vi "Lab Panel V4.83.vi"() -> ()   [LabVIEW 2013] (continued)
                n1623 = property on="SET LAB03-2" class="Clust (strict)"("DisabledEnum"=w2555) -> ()  [unwired: 2 in, 2 out]
                n1624 = property on="SET LAB04-1" class="Clust (strict)"("DisabledEnum"=w2554) -> ()  [unwired: 2 in, 2 out]
                n1625 = property on="SET LAB04-2" class="Clust (strict)"("DisabledEnum"=w2553) -> ()  [unwired: 2 in, 2 out]
                n1626 = property on="O/I  LAB05-2" class="Bool (strict)"("DisabledEnum"=w2551) -> ()  [unwired: 2 in, 2 out]
                n1627 = property on="O/I  LAB05-1" class="Bool (strict)"("DisabledEnum"=w2552) -> ()  [unwired: 2 in, 2 out]
                n1628 = property on="O/I  LAB04-1" class="Bool (strict)"("DisabledEnum"=w2554) -> ()  [unwired: 2 in, 2 out]
                n1629 = property on="O/I  LAB04-2" class="Bool (strict)"("DisabledEnum"=w2553) -> ()  [unwired: 2 in, 2 out]
                n1630 = property on="O/I  LAB03-2" class="Bool (strict)"("DisabledEnum"=w2555) -> ()  [unwired: 2 in, 2 out]
                n1631 = Not(x=w2560) -> (.not. x?=w2561:bool)
                n1632 = Not(x=w2559) -> (.not. x?=w2562:bool)
                n1633 = Not(x=w2558) -> (.not. x?=w2563:bool)
                n1634 = property on="RESULT LAB05-2" class="Bool (strict)"("Visible"=w2561) -> ()  [unwired: 2 in, 2 out]
                n1635 = property on="RESULT LAB05-1" class="Bool (strict)"("Visible"=w2562) -> ()  [unwired: 2 in, 2 out]
                n1636 = Not(x=w2557) -> (.not. x?=w2564:bool)
                n1637 = property on="RESULT LAB04-2" class="Bool (strict)"("Visible"=w2563) -> ()  [unwired: 2 in, 2 out]
                n1638 = Not(x=w2556) -> (.not. x?=w2565:bool)
                n1639 = property on="RESULT LAB04-1" class="Bool (strict)"("Visible"=w2564) -> ()  [unwired: 2 in, 2 out]
                n1640 = property on="RESULT LAB03-2" class="Bool (strict)"("Visible"=w2565) -> ()  [unwired: 2 in, 2 out]
              }
              frame #2 {
                # "disable calibrate if any test running"
                n1641 = Or(x=w2588, y=w2587) -> (x .or. y?=w2581:bool)
                n1642 = Or(x=w2590, y=w2589) -> (x .or. y?=w2583:bool)
                n1643 = Or(x=w2594, y=w2593) -> (x .or. y?=w2585:bool)
                n1644 = Or(x=w2592, y=w2591) -> (x .or. y?=w2584:bool)
                n1645 = Or(x=w2596, y=w2595) -> (x .or. y?=w2586:bool)
                n1646 = Or(x=w2584, y=w2583) -> (x .or. y?=w2582:bool)
                n1647 = Or(x=w2586, y=w2585) -> (x .or. y?=w2580:bool)
                n1648 = Or(x=w2582, y=w2581) -> (x .or. y?=w2579:bool)
                n1649 = Or(x=w2580, y=w2579) -> (x .or. y?=w2578:bool)
                n1650 = case shown="False" w2578 {
                  tunnel: [0 2] -> w2577
                  frame False {
                  }
                  frame True {
                  }
                }
                n1651 = property on="JIG TEST" class="Clust (strict)"("DisabledEnum"=w2577) -> ()  [unwired: 2 in, 2 out]
                n1652 = property on="Network Directory" class="Path"("DisabledEnum"=w2577) -> ()  [unwired: 2 in, 2 out]
                n1653 = property on="MAIL SETTINGS" class="Clust (strict)"("DisabledEnum"=w2577) -> ()  [unwired: 2 in, 2 out]
                n1654 = property on="SET (cal)" class="Bool (strict)"("DisabledEnum"=w2577) -> ()  [unwired: 2 in, 2 out]
                n1655 = property on="ADMIN" class="Bool (strict)"("DisabledEnum"=0) -> ()  [unwired: 2 in, 2 out]
              }
            }
          }
          frame #8 {
            # "drive jigs"
            n1656 = stacked-sequence {
              frame #0 {
                # "jig on"
                n1657 = local read "jig cycle"() -> (w2604:dbl)
                n1658 = property on="JIG TEST" class="Clust (strict)"() -> ("DisabledEnum"=w2601:T14)  [unwired: 2 in, 2 out]
                n1659 = Equal?(x=w2601, y=2) -> (x = y?=w2600:bool)
                n1660 = Equal?(x=w2604, y=0) -> (x = y?=w2602:bool)
                n1661 = And(x=w2602, y=w2600) -> (x .and. y?=w2599:bool)
                n1662 = case shown="True" w2599 {
                  frame False {
                  }
                  frame True {
                    n1663 = local read "run lab01-1"() -> (w2615:bool)
                    n1664 = local read "run lab01-2"() -> (w2614:bool)
                    n1665 = local read "run lab02-1"() -> (w2613:bool)
                    n1666 = local read "run lab02-2"() -> (w2612:bool)
                    n1667 = local read "run lab03-1"() -> (w2611:bool)
                    n1668 = local read "run lab03-2"() -> (w2610:bool)
                    n1669 = local read "run lab04-1"() -> (w2609:bool)
                    n1670 = local read "run lab04-2"() -> (w2608:bool)
                    n1671 = local read "run lab05-1"() -> (w2607:bool)
                    n1672 = local read "run lab05-2"() -> (w2606:bool)
                    n1673 = local write "JIG LAB03-2"(w2610) -> ()
                    n1674 = local write "JIG LAB01-1"(w2615) -> ()
                    n1675 = local write "JIG LAB01-2"(w2614) -> ()
                    n1676 = local write "JIG LAB02-1"(w2613) -> ()
                    n1677 = local write "JIG LAB02-2"(w2612) -> ()
                    n1678 = local write "JIG LAB03-1"(w2611) -> ()
                    n1679 = local write "JIG LAB04-1"(w2609) -> ()
                    n1680 = local write "JIG LAB04-2"(w2608) -> ()
                    n1681 = local write "JIG LAB05-1"(w2607) -> ()
                    n1682 = local write "JIG LAB05-2"(w2606) -> ()
                  }
                }
              }
              frame #1 {
                # "jig off"
                n1683 = local read "jig cycle"() -> (w2622:dbl)
                n1684 = local read "on loops"() -> (w2621:dbl)
                n1685 = property on="JIG TEST" class="Clust (strict)"() -> ("DisabledEnum"=w2620:T14)  [unwired: 2 in, 2 out]
                n1686 = Equal?(x=w2620, y=2) -> (x = y?=w2618:bool)
                n1687 = Equal?(x=w2622, y=w2621) -> (x = y?=w2617:bool)
                n1688 = And(x=w2617, y=w2618) -> (x .and. y?=w2616:bool)
                n1689 = case shown="True" w2616 {
                  frame False {
                  }
                  frame True {
                    w2673 = FALSE
                    w2674 = TRUE
                    w2672 = 2
                    n1690 = local read "SELECT LAB05-2"() -> (w2663:T3)
                    n1691 = local read "SELECT LAB04-2"() -> (w2665:T3)
                    n1692 = local read "SELECT LAB04-1"() -> (w2666:T3)
                    n1693 = local read "SELECT LAB05-1"() -> (w2664:T3)
                    n1694 = local read "SELECT LAB03-2"() -> (w2667:T3)
                    n1695 = local read "SELECT LAB02-1"() -> (w2670:T3)
                    n1696 = local read "SELECT LAB03-1"() -> (w2668:T3)
                    n1697 = local read "SELECT LAB02-2"() -> (w2669:T3)
                    n1698 = local read "SELECT LAB01-2"() -> (w2671:T3)
                    n1699 = local read "run lab05-1"() -> (w2633:bool)
                    n1700 = local read "run lab05-2"() -> (w2632:bool)
                    n1701 = local read "SELECT LAB01-1"() -> (w2675:T3)
                    n1702 = local read "run lab04-2"() -> (w2634:bool)
                    n1703 = local read "run lab04-1"() -> (w2635:bool)
                    n1704 = local read "run lab01-1"() -> (w2651:bool)
                    n1705 = local read "run lab01-2"() -> (w2640:bool)
                    n1706 = local read "run lab03-2"() -> (w2636:bool)
                    n1707 = local read "run lab03-1"() -> (w2637:bool)
                    n1708 = local read "run lab02-1"() -> (w2639:bool)
                    n1709 = local read "run lab02-2"() -> (w2638:bool)
                    n1710 = Equal?(x=w2672, y=w2668) -> (x = y?=w2646:bool)
                    n1711 = Equal?(x=w2672, y=w2667) -> (x = y?=w2645:bool)
                    n1712 = Equal?(x=w2672, y=w2666) -> (x = y?=w2644:bool)
                    n1713 = Equal?(x=w2672, y=w2665) -> (x = y?=w2643:bool)
                    n1714 = Equal?(x=w2672, y=w2664) -> (x = y?=w2642:bool)
                    n1715 = Equal?(x=w2672, y=w2663) -> (x = y?=w2641:bool)
                    n1716 = Equal?(x=w2672, y=w2675) -> (x = y?=w2652:bool)
                    n1717 = Equal?(x=w2672, y=w2670) -> (x = y?=w2648:bool)
                    n1718 = Equal?(x=w2672, y=w2669) -> (x = y?=w2647:bool)
                    n1719 = Equal?(x=w2672, y=w2671) -> (x = y?=w2649:bool)
                    n1720 = And(x=w2643, y=w2634) -> (x .and. y?=w2625:bool)
                    n1721 = And(x=w2646, y=w2637) -> (x .and. y?=w2628:bool)
                    n1722 = And(x=w2644, y=w2635) -> (x .and. y?=w2626:bool)
                    n1723 = And(x=w2641, y=w2632) -> (x .and. y?=w2623:bool)
                    n1724 = And(x=w2647, y=w2638) -> (x .and. y?=w2629:bool)
                    n1725 = And(x=w2645, y=w2636) -> (x .and. y?=w2627:bool)
                    n1726 = And(x=w2642, y=w2633) -> (x .and. y?=w2624:bool)
                    n1727 = And(x=w2649, y=w2640) -> (x .and. y?=w2631:bool)
                    n1728 = And(x=w2652, y=w2651) -> (x .and. y?=w2650:bool)
                    n1729 = And(x=w2648, y=w2639) -> (x .and. y?=w2630:bool)
                    n1730 = Select(t=w2674, s=w2650, f=w2673) -> (s? t:f=w2653:bool)
                    n1731 = Select(t=w2674, s=w2631, f=w2673) -> (s? t:f=w2654:bool)
                    n1732 = Select(t=w2674, s=w2630, f=w2673) -> (s? t:f=w2655:bool)
                    n1733 = Select(t=w2674, s=w2629, f=w2673) -> (s? t:f=w2656:bool)
                    n1734 = Select(t=w2674, s=w2628, f=w2673) -> (s? t:f=w2657:bool)
                    n1735 = Select(t=w2674, s=w2627, f=w2673) -> (s? t:f=w2658:bool)
                    n1736 = Select(t=w2674, s=w2626, f=w2673) -> (s? t:f=w2659:bool)
                    n1737 = Select(t=w2674, s=w2625, f=w2673) -> (s? t:f=w2660:bool)
                    n1738 = Select(t=w2674, s=w2624, f=w2673) -> (s? t:f=w2661:bool)
                    n1739 = Select(t=w2674, s=w2623, f=w2673) -> (s? t:f=w2662:bool)
                    n1740 = local write "JIG LAB03-2"(w2658) -> ()
                    n1741 = local write "JIG LAB02-1"(w2655) -> ()
                    n1742 = local write "JIG LAB02-2"(w2656) -> ()
                    n1743 = local write "JIG LAB01-2"(w2654) -> ()
                    n1744 = local write "JIG LAB03-1"(w2657) -> ()
                    n1745 = local write "JIG LAB01-1"(w2653) -> ()
                    n1746 = local write "JIG LAB05-2"(w2662) -> ()
                    n1747 = local write "JIG LAB04-1"(w2659) -> ()
                    n1748 = local write "JIG LAB05-1"(w2661) -> ()
                    n1749 = local write "JIG LAB04-2"(w2660) -> ()
                  }
                }
              }
            }
          }
          frame #9 {
            # "enable  jig test output if no test busy"
            n1750 = property on="JIG TEST" class="Clust (strict)"() -> ("DisabledEnum"=w2678:T14)  [unwired: 2 in, 2 out]
            n1751 = Equal?(x=w2678, y=0) -> (x = y?=w2676:bool)
            n1752 = case shown="True" w2676 {
              frame False {
              }
              frame True {
                n1753 = local read "JIG TEST"() -> (w2689:T9)
                n1754 = Unbundle(w2689) -> ("LAB01-1"=w2688:bool, "LAB01-2"=w2687:bool, "LAB02-1"=w2686:bool, "LAB02-2"=w2685:bool, "LAB03-1"=w2684:bool, "LAB03-2"=w2683:bool, "LAB04-1"=w2682:bool, "LAB04-2"=w2681:bool, "LAB05-1"=w2680:bool, "LAB05-2"=w2679:bool)
                n1755 = local write "JIG LAB05-1"(w2680) -> ()
                n1756 = local write "JIG LAB05-2"(w2679) -> ()
                n1757 = local write "JIG LAB04-1"(w2682) -> ()
                n1758 = local write "JIG LAB04-2"(w2681) -> ()
                n1759 = local write "JIG LAB03-2"(w2683) -> ()
                n1760 = local write "JIG LAB01-1"(w2688) -> ()
                n1761 = local write "JIG LAB02-1"(w2686) -> ()
                n1762 = local write "JIG LAB03-1"(w2684) -> ()
                n1763 = local write "JIG LAB01-2"(w2687) -> ()
                n1764 = local write "JIG LAB02-2"(w2685) -> ()
              }
            }
          }
          frame #10 {
            # "drive digital output"
            n1765 = local read "O/I  LAB05-2"() -> (w2696:bool)
            n1766 = local read "O/I  LAB05-1"() -> (w2698:bool)
            n1767 = local read "JIG LAB05-2"() -> (w2695:bool)
            n1768 = local read "O/I  LAB04-2"() -> (w2700:bool)
            n1769 = local read "JIG LAB05-1"() -> (w2697:bool)
            n1770 = local read "JIG LAB04-2"() -> (w2699:bool)
            n1771 = local read "O/I  LAB03-1"() -> (w2705:bool)
            n1772 = local read "O/I  LAB04-1"() -> (w2701:bool)
            n1773 = local read "O/I  LAB02-1"() -> (w2709:bool)
            n1774 = local read "O/I  LAB02-2"() -> (w2707:bool)
            n1775 = local read "O/I  LAB03-2"() -> (w2703:bool)
            n1776 = local read "JIG LAB04-1"() -> (w2694:bool)
            n1777 = local read "JIG LAB03-2"() -> (w2702:bool)
            n1778 = local read "O/I  LAB01-2"() -> (w2711:bool)
            n1779 = local read "JIG LAB02-1"() -> (w2708:bool)
            n1780 = local read "JIG LAB02-2"() -> (w2706:bool)
            n1781 = local read "JIG LAB03-1"() -> (w2704:bool)
            n1782 = local read "O/I  LAB01-1"() -> (w2713:bool)
            n1783 = local read "JIG LAB01-2"() -> (w2710:bool)
            n1784 = local read "JIG LAB01-1"() -> (w2712:bool)
            n1785 = Build Array(w2700, w2699, w2698, w2697, w2696, w2695) -> (w2691:bool[])
            n1786 = Build Array(w2706, w2705, w2704, w2703, w2702, w2701, w2694) -> (w2692:bool[])
            n1787 = Build Array(w2713, w2712, w2711, w2710, w2709, w2708, w2707) -> (w2693:bool[])
            n1788 = local read "simulate"() -> (w2690:bool)
            n1789 = case shown="False" w2690 {
              tunnel: w2693 -> [w2716 _]
              tunnel: w2692 -> [w2715 _]
              tunnel: w2691 -> [w2714 _]
              frame False {
                n1790 = call "sub vi - Drive Relays All v6.vi"("Array #2"=w2714, "Array #1"=w2715, "Array #0"=w2716) -> ()  [unwired: 8 in, 1 out]
              }
              frame True {
              }
            }
          }
          frame #11 {
            # "get analog values"
            n1791 = local read "on loops"() -> (w2723:dbl)
            n1792 = local read "jig cycle"() -> (w2720:dbl)
            n1793 = Add(x=w2723, y=1) -> (x+y=w2721:dbl)
            n1794 = Equal?(x=w2720, y=1) -> (x = y?=w2718:bool)
            n1795 = Equal?(x=w2720, y=w2721) -> (x = y?=w2719:bool)
            n1796 = Or(x=w2718, y=w2719) -> (x .or. y?=w2717:bool)
            n1797 = case shown="True" w2717 {
              frame False {
              }
              frame True {
                n1798 = local read "simulate"() -> (w2727:bool)
                n1799 = case shown="False" w2727 {
                  tunnel: [w2743 errorcluster[] [] ("array ERROR")] -> w2735
                  tunnel: [w2742 0.3 ("Analog loop time")] -> w2734
                  tunnel: [w2741 dynamicdata[] [] ("array GRAPH")] -> w2733
                  tunnel: [w2740 w2745] -> w2732
                  tunnel: [w2739 w2745] -> w2731
                  tunnel: [w2738 w2745] -> w2730
                  tunnel: [w2737 w2745] -> w2729
                  tunnel: [w2736 w2745] -> w2728
                  frame False {
                    n1800 = call "sub vi - Read Analog All v8.vi"() -> ("Analog loop time"=w2742:dbl, "array GRAPH"=w2741:dynamicdata[], "LAB01"=w2740:T23, "LAB02"=w2739:T24, "LAB03"=w2738:T25, "LAB04"=w2737:T26, "array ERROR"=w2743:errorcluster[], "LAB05"=w2736:T27)  [unwired: 8 in]
                  }
                  frame True {
                    w2745 = T27 {"LAB05-1 (A)"=10.0, "LAB05-1 (V)"=220.0, "LAB05-1 (PF)"=0.5, "LAB05-2 (A)"=15.0, "LAB05-2 (V)"=225.0, "LAB05-2 (PF)"=0.6} ("LAB05")
                  }
                }
                n1801 = local read "simulate"() -> (w2726:bool)
                n1802 = stacked-sequence {
                  tunnel: w2735 -> [w2752 _ _ _ _ _]
                  tunnel: w2734 -> [w2751 _ _ _ _ _]
                  tunnel: w2733 -> [w2750 _ _ _ _ _]
                  tunnel: w2732 -> [_ w2799 _ _ _ _]
                  tunnel: w2731 -> [_ _ w2806 _ _ _]
                  tunnel: w2730 -> [_ _ _ w2835 _ _]
                  tunnel: w2729 -> [_ _ _ _ w2862 _]
                  tunnel: w2728 -> [_ _ _ _ _ w2891]
                  tunnel: w2726 -> [_ w2777 w2805 w2833 w2861 w2889]
                  tunnel: T12 {"1  (A) cal"=1.0, "1 (V) cal"=1.0, "1 (PF) cal"=1.0, "1 (TL) cal"=1.0, "1 (TN) cal"=1.0, "2 (A) cal"=1.0, "2 (V) cal"=1.0, "2 (PF) cal"=1.0, "2 (TL) cal"=1.0, "2 (TN) cal"=1.0} ("CAL LAB01") -> [_ w2776 w2804 w2832 w2860 w2888]
                  frame #0 {
                    n1803 = local write "AI"(TRUE) -> ()
                    n1804 = global write "Global 1.vi" "RATE(Hz)"("RATE (Hz)") -> ()
                    n1805 = global write "Global 1.vi" "SAMPLES"("SAMPLES") -> ()
                    n1806 = Index Array(array=w2750, index=6) -> (element=→"LAB04-1 (GRAPH)":dynamicdata)
                    n1807 = Index Array(array=w2750, index=7) -> (element=→"LAB04-2 (GRAPH)":dynamicdata)
                    n1808 = Index Array(array=w2750, index=9) -> (element=→"LAB05-2 (GRAPH)":dynamicdata)
                    n1809 = Index Array(array=w2750, index=8) -> (element=→"LAB05-1 (GRAPH)":dynamicdata)
                    n1810 = Index Array(array=w2750, index=5) -> (element=→"LAB03-2 (GRAPH)":dynamicdata)
                    n1811 = Index Array(array=w2750, index=0) -> (element=→"LAB01-1 (GRAPH)":dynamicdata)
                    n1812 = Index Array(array=w2750, index=1) -> (element=→"LAB01-2 (GRAPH)":dynamicdata)
                    n1813 = Index Array(array=w2750, index=2) -> (element=→"LAB02-1 (GRAPH)":dynamicdata)
                    n1814 = Index Array(array=w2750, index=3) -> (element=→"LAB02-2 (GRAPH)":dynamicdata)
                    n1815 = Index Array(array=w2750, index=4) -> (element=→"LAB03-1 (GRAPH)":dynamicdata)
                    "AI loop time" <- w2751
                    "Analog Error Array" <- w2752
                  }
                  frame #1 {
                    n1816 = Unbundle By Name(w2799) -> ("LAB05-1 (A)"=w2797:dbl, "LAB05-1 (V)"=w2796:dbl, "LAB05-1 (PF)"=w2795:dbl, "LAB05-2 (A)"=w2794:dbl, "LAB05-2 (V)"=w2793:dbl, "LAB05-2 (PF)"=w2792:dbl)
                    n1817 = case shown="False" w2777 {
                      tunnel: [w2800 w2801] -> w2798
                      tunnel: w2776 -> [_ w2801]
                      frame False {
                        n1818 = local read "CAL LAB01"() -> (w2800:T12)
                      }
                      frame True {
                      }
                    }
                    n1819 = Unbundle By Name(w2798) -> ("1  (A) cal"=w2791:dbl, "1 (V) cal"=w2790:dbl, "1 (PF) cal"=w2789:dbl, "2 (A) cal"=w2788:dbl, "2 (V) cal"=w2787:dbl, "2 (PF) cal"=w2786:dbl)  [unwired: 4 out]
                    n1820 = Multiply(x=w2797, y=w2791) -> (x*y=w2784:dbl)
                    n1821 = Multiply(x=w2796, y=w2790) -> (x*y=w2783:dbl)
                    n1822 = Multiply(x=w2795, y=w2789) -> (x*y=w2782:dbl)
                    n1823 = Multiply(x=w2794, y=w2788) -> (x*y=w2780:dbl)
                    n1824 = Multiply(x=w2793, y=w2787) -> (x*y=w2779:dbl)
                    n1825 = Multiply(x=w2792, y=w2786) -> (x*y=w2778:dbl)
                    n1826 = local read "SIG LAB01-1"() -> (w2785:T2)
                    n1827 = local read "SIG LAB01-2"() -> (w2781:T2)
                    n1828 = Bundle By Name(cluster=w2785, "AMPS"=w2784, "VOLTS"=w2783, "PF"=w2782) -> (w2775:T2)
                    n1829 = Bundle By Name(cluster=w2781, "AMPS"=w2780, "VOLTS"=w2779, "PF"=w2778) -> (w2774:T2)
                    n1830 = global write "Global display 1.vi" "SIG LAB01-2"(w2774) -> ()
                    n1831 = global write "Global display 1.vi" "SIG LAB01-1"(w2775) -> ()
                    n1832 = local write "SIG LAB01-2"(w2774) -> ()
                    n1833 = local write "SIG LAB01-1"(w2775) -> ()
                  }
                  frame #2 {
                    n1834 = Unbundle By Name(w2806) -> ("LAB05-1 (A)"=w2826:dbl, "LAB05-1 (V)"=w2825:dbl, "LAB05-1 (PF)"=w2824:dbl, "LAB05-2 (A)"=w2823:dbl, "LAB05-2 (V)"=w2822:dbl, "LAB05-2 (PF)"=w2821:dbl)
                    n1835 = case shown="True" w2805 {
                      tunnel: [w2828 w2829] -> w2827
                      tunnel: w2804 -> [_ w2829]
                      frame False {
                        n1836 = local read "CAL LAB02"() -> (w2828:T13)
                      }
                      frame True {
                      }
                    }
                    n1837 = Unbundle By Name(w2827) -> ("1  (A) cal"=w2820:dbl, "1 (V) cal"=w2819:dbl, "1 (PF) cal"=w2818:dbl, "2 (A) cal"=w2817:dbl, "2 (V) cal"=w2816:dbl, "2 (PF) cal"=w2815:dbl)  [unwired: 4 out]
                    n1838 = Multiply(x=w2826, y=w2820) -> (x*y=w2813:dbl)
                    n1839 = Multiply(x=w2825, y=w2819) -> (x*y=w2812:dbl)
                    n1840 = Multiply(x=w2824, y=w2818) -> (x*y=w2811:dbl)
                    n1841 = Multiply(x=w2823, y=w2817) -> (x*y=w2809:dbl)
                    n1842 = Multiply(x=w2822, y=w2816) -> (x*y=w2808:dbl)
                    n1843 = Multiply(x=w2821, y=w2815) -> (x*y=w2807:dbl)
                    n1844 = local read "SIG LAB02-1"() -> (w2814:T2)
                    n1845 = local read "SIG LAB02-2"() -> (w2810:T2)
                    n1846 = Bundle By Name(cluster=w2814, "AMPS"=w2813, "VOLTS"=w2812, "PF"=w2811) -> (w2803:T2)
                    n1847 = Bundle By Name(cluster=w2810, "AMPS"=w2809, "VOLTS"=w2808, "PF"=w2807) -> (w2802:T2)
                    n1848 = global write "Global display 1.vi" "SIG LAB02-1"(w2803) -> ()
                    n1849 = local write "SIG LAB02-2"(w2802) -> ()
                    n1850 = global write "Global display 1.vi" "SIG LAB02-2"(w2802) -> ()
                    n1851 = local write "SIG LAB02-1"(w2803) -> ()
                  }
                  frame #3 {
                    n1852 = Unbundle By Name(w2835) -> ("LAB05-1 (A)"=w2854:dbl, "LAB05-1 (V)"=w2853:dbl, "LAB05-1 (PF)"=w2852:dbl, "LAB05-2 (A)"=w2851:dbl, "LAB05-2 (V)"=w2850:dbl, "LAB05-2 (PF)"=w2849:dbl)
                    n1853 = case shown="True" w2833 {
                      tunnel: [w2856 w2857] -> w2855
                      tunnel: w2832 -> [_ w2857]
                      frame False {
                        n1854 = local read "CAL LAB03"() -> (w2856:T12)
                      }
                      frame True {
                      }
                    }
                    n1855 = Unbundle By Name(w2855) -> ("1  (A) cal"=w2848:dbl, "1 (V) cal"=w2847:dbl, "1 (PF) cal"=w2846:dbl, "2 (A) cal"=w2845:dbl, "2 (V) cal"=w2844:dbl, "2 (PF) cal"=w2843:dbl)  [unwired: 4 out]
                    n1856 = Multiply(x=w2854, y=w2848) -> (x*y=w2841:dbl)
                    n1857 = Multiply(x=w2853, y=w2847) -> (x*y=w2834:dbl)
                    n1858 = Multiply(x=w2852, y=w2846) -> (x*y=w2840:dbl)
                    n1859 = Multiply(x=w2851, y=w2845) -> (x*y=w2838:dbl)
                    n1860 = Multiply(x=w2850, y=w2844) -> (x*y=w2837:dbl)
                    n1861 = Multiply(x=w2849, y=w2843) -> (x*y=w2836:dbl)
                    n1862 = local read "SIG LAB03-1"() -> (w2842:T2)
                    n1863 = local read "SIG LAB03-2"() -> (w2839:T2)
                    n1864 = Bundle By Name(cluster=w2842, "AMPS"=w2841, "VOLTS"=w2834, "PF"=w2840) -> (w2831:T2)
                    n1865 = Bundle By Name(cluster=w2839, "AMPS"=w2838, "VOLTS"=w2837, "PF"=w2836) -> (w2830:T2)
                    n1866 = global write "Global display 1.vi" "SIG LAB03-1"(w2831) -> ()
                    n1867 = global write "Global display 1.vi" "SIG LAB03-2"(w2830) -> ()
                    n1868 = local write "SIG LAB03-2"(w2830) -> ()
                    n1869 = local write "SIG LAB03-1"(w2831) -> ()
                  }
                  frame #4 {
                    n1870 = Unbundle By Name(w2862) -> ("LAB05-1 (A)"=w2882:dbl, "LAB05-1 (V)"=w2881:dbl, "LAB05-1 (PF)"=w2880:dbl, "LAB05-2 (A)"=w2879:dbl, "LAB05-2 (V)"=w2878:dbl, "LAB05-2 (PF)"=w2877:dbl)
                    n1871 = case shown="False" w2861 {
                      tunnel: [w2884 w2885] -> w2883
                      tunnel: w2860 -> [_ w2885]
                      frame False {
                        n1872 = local read "CAL LAB04"() -> (w2884:T12)
                      }
                      frame True {
                      }
                    }
                    n1873 = Unbundle By Name(w2883) -> ("1  (A) cal"=w2876:dbl, "1 (V) cal"=w2875:dbl, "1 (PF) cal"=w2874:dbl, "2 (A) cal"=w2873:dbl, "2 (V) cal"=w2872:dbl, "2 (PF) cal"=w2871:dbl)  [unwired: 4 out]
                    n1874 = Multiply(x=w2882, y=w2876) -> (x*y=w2869:dbl)
                    n1875 = Multiply(x=w2881, y=w2875) -> (x*y=w2868:dbl)
                    n1876 = Multiply(x=w2880, y=w2874) -> (x*y=w2867:dbl)
                    n1877 = Multiply(x=w2879, y=w2873) -> (x*y=w2865:dbl)
                    n1878 = Multiply(x=w2878, y=w2872) -> (x*y=w2864:dbl)
                    n1879 = Multiply(x=w2877, y=w2871) -> (x*y=w2863:dbl)
                    n1880 = local read "SIG LAB04-1"() -> (w2870:T2)
                    n1881 = local read "SIG LAB04-2"() -> (w2866:T2)
                    n1882 = Bundle By Name(cluster=w2870, "AMPS"=w2869, "VOLTS"=w2868, "PF"=w2867) -> (w2859:T2)
                    n1883 = Bundle By Name(cluster=w2866, "AMPS"=w2865, "VOLTS"=w2864, "PF"=w2863) -> (w2858:T2)
                    n1884 = global write "Global display 1.vi" "SIG LAB04-2"(w2858) -> ()
                    n1885 = global write "Global display 1.vi" "SIG LAB04-1"(w2859) -> ()
                    n1886 = local write "SIG LAB04-2"(w2858) -> ()
                    n1887 = local write "SIG LAB04-1"(w2859) -> ()
                  }
                  frame #5 {
                    n1888 = Unbundle By Name(w2891) -> ("LAB05-1 (A)"=w2910:dbl, "LAB05-1 (V)"=w2890:dbl, "LAB05-1 (PF)"=w2909:dbl, "LAB05-2 (A)"=w2908:dbl, "LAB05-2 (V)"=w2907:dbl, "LAB05-2 (PF)"=w2906:dbl)
                    n1889 = case shown="False" w2889 {
                      tunnel: [w2912 w2913] -> w2911
                      tunnel: w2888 -> [_ w2913]
                      frame False {
                        n1890 = local read "CAL LAB05"() -> (w2912:T12)
                      }
                      frame True {
                      }
                    }
                    n1891 = Unbundle By Name(w2911) -> ("1  (A) cal"=w2905:dbl, "1 (V) cal"=w2904:dbl, "1 (PF) cal"=w2903:dbl, "2 (A) cal"=w2902:dbl, "2 (V) cal"=w2901:dbl, "2 (PF) cal"=w2900:dbl)  [unwired: 4 out]
                    n1892 = Multiply(x=w2910, y=w2905) -> (x*y=w2898:dbl)
                    n1893 = Multiply(x=w2890, y=w2904) -> (x*y=w2897:dbl)
                    n1894 = Multiply(x=w2909, y=w2903) -> (x*y=w2896:dbl)
                    n1895 = Multiply(x=w2908, y=w2902) -> (x*y=w2894:dbl)
                    n1896 = Multiply(x=w2907, y=w2901) -> (x*y=w2893:dbl)
                    n1897 = Multiply(x=w2906, y=w2900) -> (x*y=w2892:dbl)
                    n1898 = local read "SIG LAB05-1"() -> (w2899:T2)
                    n1899 = local read "SIG LAB05-2"() -> (w2895:T2)
                    n1900 = Bundle By Name(cluster=w2899, "AMPS"=w2898, "VOLTS"=w2897, "PF"=w2896) -> (w2887:T2)
                    n1901 = Bundle By Name(cluster=w2895, "AMPS"=w2894, "VOLTS"=w2893, "PF"=w2892) -> (w2886:T2)
                    n1902 = global write "Global display 1.vi" "SIG LAB05-1"(w2887) -> ()
                    n1903 = global write "Global display 1.vi" "SIG LAB05-2"(w2886) -> ()
                    n1904 = local write "SIG LAB05-2"(w2886) -> ()
                    n1905 = local write "SIG LAB05-1"(w2887) -> ()
                  }
                }
              }
            }
          }
          frame #12 {
            # "save test data to file"
            n1906 = Get Date/Time In Seconds() -> (seconds since 1Jan1904=w2914:timestamp)
            "File Time Stamp" <- w2914
            n1907 = local read "on loops"() -> (w2933:dbl)
            n1908 = local read "jig cycle"() -> (w2930:dbl)
            n1909 = Format Date/Time String(time format string (%c)="%H:%M%:%S", seconds (now)=w2914) -> (date/time string=w2918:string)  [unwired: 1 in]
            n1910 = Add(x=w2933, y=2) -> (x+y=w2931:dbl)
            n1911 = Build Array(w2918) -> (w2917:string[])
            n1912 = Equal?(x=w2930, y=1) -> (x = y?=w2916:bool)
            n1913 = Equal?(x=w2930, y=w2931) -> (x = y?=w2915:bool)
            n1914 = stacked-sequence {
              tunnel: w2929 -> [w2939 _ _ _ _ _ _ _ _ _]
              tunnel: w2928 -> [_ w3015 _ _ _ _ _ _ _ _]
              tunnel: w2927 -> [_ _ w3095 _ _ _ _ _ _ _]
              tunnel: w2926 -> [_ _ _ w3175 _ _ _ _ _ _]
              tunnel: w2925 -> [_ _ _ _ w3255 _ _ _ _ _]
              tunnel: w2924 -> [_ _ _ _ _ w3335 _ _ _ _]
              tunnel: w2923 -> [_ _ _ _ _ _ w3415 _ _ _]
              tunnel: w2922 -> [_ _ _ _ _ _ _ w3495 _ _]
              tunnel: w2921 -> [_ _ _ _ _ _ _ _ w3575 _]
              tunnel: w2920 -> [_ _ _ _ _ _ _ _ _ w3655]
              tunnel: w2917 -> [w2938 w3019 w3099 w3179 w3259 w3339 w3419 w3499 w3579 w3659]
              tunnel: w2916 -> [w2937 w3018 w3098 w3178 w3258 w3338 w3418 w3498 w3578 w3658]
              tunnel: w2915 -> [w2936 w3017 w3097 w3177 w3257 w3337 w3417 w3497 w3577 w3657]
              tunnel: w2914 -> [w2935 w3016 w3096 w3176 w3256 w3336 w3416 w3496 w3576 w3656]
              frame #0 {
                n1915 = case shown="True" w2939 {
                  tunnel: w2938 -> [_ w2944]
                  tunnel: w2937 -> [_ w2943]
                  tunnel: w2936 -> [_ w2941]
                  tunnel: w2935 -> [_ w2940]
                  frame False {
                  }
                  frame True {
                    n1916 = local read "DISP LAB01-1"() -> (w2945:T4)
                    n1917 = local read "SIG LAB01-1"() -> (w2946:T2)
                    n1918 = local read "ON L01-1"() -> (w2942:cluster{"amps":dbl, "volts":dbl, "pf":dbl})
                    n1919 = Unbundle(w2946) -> ("AMPS"=w2952:dbl, "VOLTS"=w2950:dbl, "PF"=w2949:dbl, "Tmp Live"=w2948:dbl, "Tmp Neut"=w2951:dbl)
                    n1920 = Unbundle(w2945) -> ("CYCLE"=w2947:dbl)  [unwired: 2 out]
                    n1921 = stacked-sequence {
                      tunnel: w2952 -> [w2956 w2975]
                      tunnel: w2951 -> [_ w2974]
                      tunnel: w2950 -> [w2955 w2973]
                      tunnel: w2949 -> [w2954 w2972]
                      tunnel: w2948 -> [_ w2971]
                      tunnel: w2947 -> [_ w2970]
                      tunnel: w2944 -> [_ w2969]
                      tunnel: w2943 -> [w2957 _]
                      tunnel: w2942 -> [w2953 w2967]
                      tunnel: w2941 -> [_ w2968]
                      tunnel: w2940 -> [_ w2963]
                      frame #0 {
                        n1922 = case shown="True" w2957 {
                          tunnel: w2956 -> [_ w2962]
                          tunnel: w2955 -> [_ w2961]
                          tunnel: w2954 -> [_ w2960]
                          tunnel: w2953 -> [_ w2958]
                          frame False {
                          }
                          frame True {
                            n1923 = Bundle(cluster=w2958, "amps"=w2962, "volts"=w2961, "pf"=w2960) -> (w2959:cluster{"amps":dbl, "volts":dbl, "pf":dbl})
                            n1924 = local write "ON L01-1"(w2959) -> ()
                          }
                        }
                      }
                      frame #1 {
                        n1925 = Unbundle(w2967) -> ("amps"=w2966:dbl, "volts"=w2965:dbl, "pf"=w2964:dbl)
                        n1926 = case shown="True" w2968 {
                          tunnel: w2975 -> [_ w2976]
                          tunnel: w2974 -> [_ w3014]
                          tunnel: w2973 -> [_ _]
                          tunnel: w2972 -> [_ _]
                          tunnel: w2971 -> [_ w3013]
                          tunnel: w2970 -> [_ w3012]
                          tunnel: w2969 -> [_ w2980]
                          tunnel: w2966 -> [_ w2977]
                          tunnel: w2965 -> [_ w3009]
                          tunnel: w2964 -> [_ w3008]
                          tunnel: w2963 -> [_ w2978]
                          frame False {
                          }
                          frame True {
                            n1927 = local read "TDMS LAB01-1"() -> (w3011:refnum<k34>)
                            n1928 = Build Array(w3009) -> (w3005:dbl[])
                            n1929 = Build Array(w3008) -> (w3004:dbl[])
                            n1930 = Build Array(w3013) -> (w3003:dbl[])
                            n1931 = Build Array(w3014) -> (w3002:dbl[])
                            n1932 = Build Array(w2977) -> (w3007:dbl[])
                            n1933 = Build Array(w2976) -> (w3006:dbl[])
                            n1934 = Build Array(w3012) -> (w3001:dbl[])
                            n1935 = Build Array("AMPS ON", "AMPS OFF", "VOLTS", "PF", "TEMP Live", "TEMP Neut", "CYCLE") -> (w2985:string[])
                            n1936 = Bundle By Name("Y"=w3007, "t0"=w2978) -> (w3000:waveform(dbl))  [unwired: 1 in]
                            n1937 = Bundle By Name("Y"=w3006, "t0"=w2978) -> (w2999:waveform(dbl))  [unwired: 1 in]
                            n1938 = Bundle By Name("Y"=w3005, "t0"=w2978) -> (w2998:waveform(dbl))  [unwired: 1 in]
                            n1939 = Bundle By Name("Y"=w3004, "t0"=w2978) -> (w2997:waveform(dbl))  [unwired: 1 in]
                            n1940 = Bundle By Name("Y"=w3003, "t0"=w2978) -> (w2996:waveform(dbl))  [unwired: 1 in]
                            n1941 = Bundle By Name("Y"=w3002, "t0"=w2978) -> (w2995:waveform(dbl))  [unwired: 1 in]
                            n1942 = Bundle By Name("Y"=w3001, "t0"=w2978) -> (w2994:waveform(dbl))  [unwired: 1 in]
                            n1943 = Build Array(w3000, w2999, w2998, w2997, w2996, w2995, w2994) -> (w2993:waveform(dbl)[])
                            n1944 = TDMS Write(0:w3011, 5:"TEST VALUES", 7:w2985, 9:w2993) -> (4:w2984:refnum<k34>, 6:w2983:string, 15:w2982:errorcluster)  [unwired: 2 in, 1 out]
                            n1945 = TDMS Write(0:w2984, 5:w2983, 7:"TIME", 9:w2980, 11:w2982) -> (15:w2979:errorcluster)  [unwired: 1 in, 3 out]
                            n1946 = local write "data file error"(w2979) -> ()
                          }
                        }
                      }
                    }
                  }
                }
              }
              frame #1 {
                n1947 = case shown="True" w3015 {
                  tunnel: w3019 -> [_ w3024]
                  tunnel: w3018 -> [_ w3023]
                  tunnel: w3017 -> [_ w3021]
                  tunnel: w3016 -> [_ w3020]
                  frame False {
                  }
                  frame True {
                    n1948 = local read "DISP LAB01-2"() -> (w3025:T4)
                    n1949 = local read "SIG LAB01-2"() -> (w3026:T2)
                    n1950 = local read "ON L01-2"() -> (w3022:cluster{"amps":dbl, "volts":dbl, "pf":dbl})
                    n1951 = Unbundle(w3026) -> ("AMPS"=w3032:dbl, "VOLTS"=w3030:dbl, "PF"=w3029:dbl, "Tmp Live"=w3028:dbl, "Tmp Neut"=w3031:dbl)
                    n1952 = Unbundle(w3025) -> ("CYCLE"=w3027:dbl)  [unwired: 2 out]
                    n1953 = stacked-sequence {
                      tunnel: w3032 -> [w3036 w3055]
                      tunnel: w3031 -> [_ w3054]
                      tunnel: w3030 -> [w3035 w3053]
                      tunnel: w3029 -> [w3034 w3052]
                      tunnel: w3028 -> [_ w3051]
                      tunnel: w3027 -> [_ w3050]
                      tunnel: w3024 -> [_ w3049]
                      tunnel: w3023 -> [w3037 _]
                      tunnel: w3022 -> [w3033 w3047]
                      tunnel: w3021 -> [_ w3048]
                      tunnel: w3020 -> [_ w3043]
                      frame #0 {
                        n1954 = case shown="True" w3037 {
                          tunnel: w3036 -> [_ w3042]
                          tunnel: w3035 -> [_ w3041]
                          tunnel: w3034 -> [_ w3040]
                          tunnel: w3033 -> [_ w3038]
                          frame False {
                          }
                          frame True {
                            n1955 = Bundle(cluster=w3038, "amps"=w3042, "volts"=w3041, "pf"=w3040) -> (w3039:cluster{"amps":dbl, "volts":dbl, "pf":dbl})
                            n1956 = local write "ON L01-2"(w3039) -> ()
                          }
                        }
                      }
                      frame #1 {
                        n1957 = Unbundle(w3047) -> ("amps"=w3046:dbl, "volts"=w3045:dbl, "pf"=w3044:dbl)
                        n1958 = case shown="True" w3048 {
                          tunnel: w3055 -> [_ w3087]
                          tunnel: w3054 -> [_ w3094]
                          tunnel: w3053 -> [_ _]
                          tunnel: w3052 -> [_ _]
                          tunnel: w3051 -> [_ w3093]
                          tunnel: w3050 -> [_ w3092]
                          tunnel: w3049 -> [_ w3057]
                          tunnel: w3046 -> [_ w3089]
                          tunnel: w3045 -> [_ w3088]
                          tunnel: w3044 -> [_ w3086]
                          tunnel: w3043 -> [_ w3078]
                          frame False {
                          }
                          frame True {
                            n1959 = local read "TDMS LAB01-2"() -> (w3091:refnum<k34>)
                            n1960 = Build Array(w3088) -> (w3083:dbl[])
                            n1961 = Build Array(w3086) -> (w3082:dbl[])
                            n1962 = Build Array(w3093) -> (w3081:dbl[])
                            n1963 = Build Array(w3094) -> (w3080:dbl[])
                            n1964 = Build Array(w3089) -> (w3085:dbl[])
                            n1965 = Build Array(w3087) -> (w3084:dbl[])
                            n1966 = Build Array(w3092) -> (w3079:dbl[])
                            n1967 = Build Array("AMPS ON", "AMPS OFF", "VOLTS", "PF", "TEMP Live", "TEMP Neut", "CYCLE") -> (w3062:string[])
                            n1968 = Bundle By Name("Y"=w3085, "t0"=w3078) -> (w3077:waveform(dbl))  [unwired: 1 in]
                            n1969 = Bundle By Name("Y"=w3084, "t0"=w3078) -> (w3076:waveform(dbl))  [unwired: 1 in]
                            n1970 = Bundle By Name("Y"=w3083, "t0"=w3078) -> (w3075:waveform(dbl))  [unwired: 1 in]
                            n1971 = Bundle By Name("Y"=w3082, "t0"=w3078) -> (w3074:waveform(dbl))  [unwired: 1 in]
                            n1972 = Bundle By Name("Y"=w3081, "t0"=w3078) -> (w3073:waveform(dbl))  [unwired: 1 in]
                            n1973 = Bundle By Name("Y"=w3080, "t0"=w3078) -> (w3072:waveform(dbl))  [unwired: 1 in]
                            n1974 = Bundle By Name("Y"=w3079, "t0"=w3078) -> (w3071:waveform(dbl))  [unwired: 1 in]
                            n1975 = Build Array(w3077, w3076, w3075, w3074, w3073, w3072, w3071) -> (w3070:waveform(dbl)[])
                            n1976 = TDMS Write(0:w3091, 5:"TEST VALUES", 7:w3062, 9:w3070) -> (4:w3061:refnum<k34>, 6:w3060:string, 15:w3059:errorcluster)  [unwired: 2 in, 1 out]
                            n1977 = TDMS Write(0:w3061, 5:w3060, 7:"TIME", 9:w3057, 11:w3059) -> (15:w3056:errorcluster)  [unwired: 1 in, 3 out]
                            n1978 = local write "data file error"(w3056) -> ()
                          }
                        }
                      }
                    }
                  }
                }
              }
              frame #2 {
                n1979 = case shown="True" w3095 {
                  tunnel: w3099 -> [_ w3104]
                  tunnel: w3098 -> [_ w3103]
                  tunnel: w3097 -> [_ w3101]
                  tunnel: w3096 -> [_ w3100]
                  frame False {
                  }
                  frame True {
                    n1980 = local read "DISP LAB02-1"() -> (w3105:T4)
                    n1981 = local read "SIG LAB02-1"() -> (w3106:T2)
                    n1982 = local read "ON L02-1"() -> (w3102:cluster{"amps":dbl, "volts":dbl, "pf":dbl})
                    n1983 = Unbundle(w3106) -> ("AMPS"=w3112:dbl, "VOLTS"=w3110:dbl, "PF"=w3109:dbl, "Tmp Live"=w3108:dbl, "Tmp Neut"=w3111:dbl)
                    n1984 = Unbundle(w3105) -> ("CYCLE"=w3107:dbl)  [unwired: 2 out]
                    n1985 = stacked-sequence {
                      tunnel: w3112 -> [w3116 w3135]
                      tunnel: w3111 -> [_ w3134]
                      tunnel: w3110 -> [w3115 w3133]
                      tunnel: w3109 -> [w3114 w3132]
                      tunnel: w3108 -> [_ w3131]
                      tunnel: w3107 -> [_ w3130]
                      tunnel: w3104 -> [_ w3129]
                      tunnel: w3103 -> [w3117 _]
                      tunnel: w3102 -> [w3113 w3127]
                      tunnel: w3101 -> [_ w3128]
                      tunnel: w3100 -> [_ w3123]
                      frame #0 {
                        n1986 = case shown="True" w3117 {
                          tunnel: w3116 -> [_ w3122]
                          tunnel: w3115 -> [_ w3121]
                          tunnel: w3114 -> [_ w3120]
                          tunnel: w3113 -> [_ w3118]
                          frame False {
                          }
                          frame True {
                            n1987 = Bundle(cluster=w3118, "amps"=w3122, "volts"=w3121, "pf"=w3120) -> (w3119:cluster{"amps":dbl, "volts":dbl, "pf":dbl})
                            n1988 = local write "ON L02-1"(w3119) -> ()
                          }
                        }
                      }
                      frame #1 {
                        n1989 = Unbundle(w3127) -> ("amps"=w3126:dbl, "volts"=w3125:dbl, "pf"=w3124:dbl)
                        n1990 = case shown="True" w3128 {
                          tunnel: w3135 -> [_ w3167]
                          tunnel: w3134 -> [_ w3174]
                          tunnel: w3133 -> [_ _]
                          tunnel: w3132 -> [_ _]
                          tunnel: w3131 -> [_ w3173]
                          tunnel: w3130 -> [_ w3172]
                          tunnel: w3129 -> [_ w3137]
                          tunnel: w3126 -> [_ w3169]
                          tunnel: w3125 -> [_ w3168]
                          tunnel: w3124 -> [_ w3166]
                          tunnel: w3123 -> [_ w3158]
                          frame False {
                          }
                          frame True {
                            n1991 = local read "TDMS LAB02-1"() -> (w3171:refnum<k34>)
                            n1992 = Build Array(w3168) -> (w3163:dbl[])
                            n1993 = Build Array(w3166) -> (w3162:dbl[])
                            n1994 = Build Array(w3173) -> (w3161:dbl[])
                            n1995 = Build Array(w3174) -> (w3160:dbl[])
                            n1996 = Build Array(w3169) -> (w3165:dbl[])
                            n1997 = Build Array(w3167) -> (w3164:dbl[])
                            n1998 = Build Array(w3172) -> (w3159:dbl[])
                            n1999 = Build Array("AMPS ON", "AMPS OFF", "VOLTS", "PF", "TEMP Live", "TEMP Neut", "CYCLE") -> (w3142:string[])
                            n2000 = Bundle By Name("Y"=w3165, "t0"=w3158) -> (w3157:waveform(dbl))  [unwired: 1 in]
                            n2001 = Bundle By Name("Y"=w3164, "t0"=w3158) -> (w3156:waveform(dbl))  [unwired: 1 in]
                            n2002 = Bundle By Name("Y"=w3163, "t0"=w3158) -> (w3155:waveform(dbl))  [unwired: 1 in]
                            n2003 = Bundle By Name("Y"=w3162, "t0"=w3158) -> (w3154:waveform(dbl))  [unwired: 1 in]
                            n2004 = Bundle By Name("Y"=w3161, "t0"=w3158) -> (w3153:waveform(dbl))  [unwired: 1 in]
                            n2005 = Bundle By Name("Y"=w3160, "t0"=w3158) -> (w3152:waveform(dbl))  [unwired: 1 in]
                            n2006 = Bundle By Name("Y"=w3159, "t0"=w3158) -> (w3151:waveform(dbl))  [unwired: 1 in]
                            n2007 = Build Array(w3157, w3156, w3155, w3154, w3153, w3152, w3151) -> (w3150:waveform(dbl)[])
                            n2008 = TDMS Write(0:w3171, 5:"TEST VALUES", 7:w3142, 9:w3150) -> (4:w3141:refnum<k34>, 6:w3140:string, 15:w3139:errorcluster)  [unwired: 2 in, 1 out]
                            n2009 = TDMS Write(0:w3141, 5:w3140, 7:"TIME", 9:w3137, 11:w3139) -> (15:w3136:errorcluster)  [unwired: 1 in, 3 out]
                            n2010 = local write "data file error"(w3136) -> ()
                          }
                        }
                      }
                    }
                  }
                }
              }
              frame #3 {
                n2011 = case shown="True" w3175 {
                  tunnel: w3179 -> [_ w3184]
                  tunnel: w3178 -> [_ w3183]
                  tunnel: w3177 -> [_ w3181]
                  tunnel: w3176 -> [_ w3180]
                  frame False {
                  }
                  frame True {
                    n2012 = local read "DISP LAB02-2"() -> (w3185:T4)
                    n2013 = local read "SIG LAB02-2"() -> (w3186:T2)
                    n2014 = local read "ON L02-2"() -> (w3182:cluster{"amps":dbl, "volts":dbl, "pf":dbl})
                    n2015 = Unbundle(w3186) -> ("AMPS"=w3192:dbl, "VOLTS"=w3190:dbl, "PF"=w3189:dbl, "Tmp Live"=w3188:dbl, "Tmp Neut"=w3191:dbl)
                    n2016 = Unbundle(w3185) -> ("CYCLE"=w3187:dbl)  [unwired: 2 out]
                    n2017 = stacked-sequence {
                      tunnel: w3192 -> [w3196 w3215]
                      tunnel: w3191 -> [_ w3214]
                      tunnel: w3190 -> [w3195 w3213]
                      tunnel: w3189 -> [w3194 w3212]
                      tunnel: w3188 -> [_ w3211]
                      tunnel: w3187 -> [_ w3210]
                      tunnel: w3184 -> [_ w3209]
                      tunnel: w3183 -> [w3197 _]
                      tunnel: w3182 -> [w3193 w3207]
                      tunnel: w3181 -> [_ w3208]
                      tunnel: w3180 -> [_ w3203]
                      frame #0 {
                        n2018 = case shown="True" w3197 {
                          tunnel: w3196 -> [_ w3202]
                          tunnel: w3195 -> [_ w3201]
                          tunnel: w3194 -> [_ w3200]
                          tunnel: w3193 -> [_ w3198]
                          frame False {
                          }
                          frame True {
                            n2019 = Bundle(cluster=w3198, "amps"=w3202, "volts"=w3201, "pf"=w3200) -> (w3199:cluster{"amps":dbl, "volts":dbl, "pf":dbl})
                            n2020 = local write "ON L02-2"(w3199) -> ()
                          }
                        }
                      }
                      frame #1 {
                        n2021 = Unbundle(w3207) -> ("amps"=w3206:dbl, "volts"=w3205:dbl, "pf"=w3204:dbl)
                        n2022 = case shown="True" w3208 {
                          tunnel: w3215 -> [_ w3247]
                          tunnel: w3214 -> [_ w3254]
                          tunnel: w3213 -> [_ _]
                          tunnel: w3212 -> [_ _]
                          tunnel: w3211 -> [_ w3253]
                          tunnel: w3210 -> [_ w3252]
                          tunnel: w3209 -> [_ w3217]
                          tunnel: w3206 -> [_ w3249]
                          tunnel: w3205 -> [_ w3248]
                          tunnel: w3204 -> [_ w3246]
                          tunnel: w3203 -> [_ w3238]
                          frame False {
                          }
                          frame True {
